vi "KN-AnnulusToArray.vi"(10 "Rectangle":T1 {"Rotation" format="%.2f"; "Left" scale=0.0..1024.0; "Right" scale=0.0..1024.0}, 11 "Annulus":T2 {"End Angle" format="%.2f"; "Start Angle" format="%.2f"; "Center X" scale=0.0..1024.0}) -> (2 "矩形":string, 3 "字符串":string)   [LabVIEW 2015]
panel:
  out "添加的数组":string[](array[string])
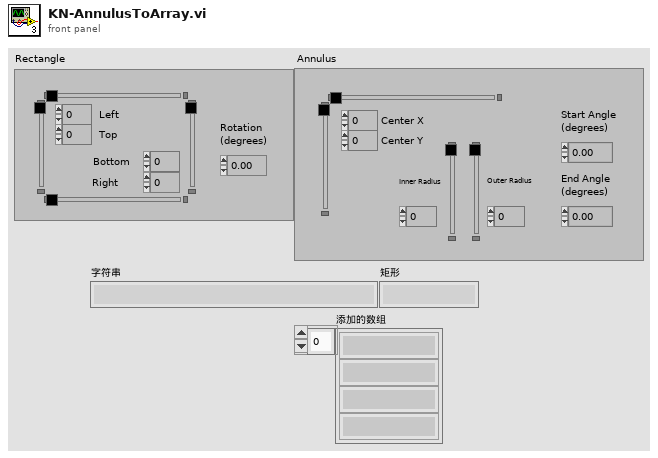
[diagram p1: front panel]
types:
  T1 = typedef "IMAQ Rectangle" = cluster{"Left":i32, "Top":i32, "Right":i32, "Bottom":i32, "Rotation":dbl}
  T2 = typedef "IMAQ Circle" = cluster{"Center X":i32, "Center Y":i32, "Inner Radius":i32, "Outer Radius":i32, "Start Angle":dbl, "End Angle":dbl}
  T3 = cluster{"Center X":string, "Center Y":string, "Inner Radius":string, "Outer Radius":string, "Start Angle":string, "End Angle":string}
  T4 = cluster{"Left":string, "Top":string, "Right":string, "Bottom":string, "Rotation":string}
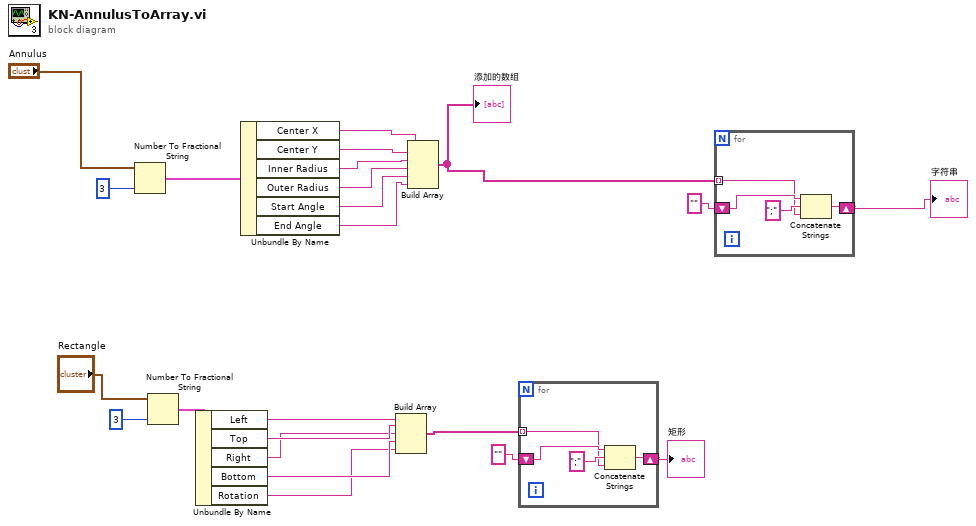
[diagram p0: block diagram]
diagram:
  n1 = Number To Fractional String(number="Annulus", precision (6)=i16 3 ("精度(6)")) -> (F-format string=w22:T3)  [unwired: 2 in]
  n2 = Number To Fractional String(number="Rectangle", precision (6)=i16 3 ("精度(6)")) -> (F-format string=w9:T4)  [unwired: 2 in]
  n3 = Unbundle By Name(w9) -> ("Left"=w8:string, "Top"=w7:string, "Right"=w6:string, "Bottom"=w5:string, "Rotation"=w4:string)
  n4 = Unbundle By Name(w22) -> ("Center X"=w21:string, "Center Y"=w20:string, "Inner Radius"=w19:string, "Outer Radius"=w18:string, "Start Angle"=w17:string, "End Angle"=w16:string)
  n5 = Build Array(w8, w7, w6, w5, w4) -> (w2:string[])
  n6 = Build Array(w21, w20, w19, w18, w17, w16) -> (w15:string[])
  "添加的数组" <- w15
  n7 = for {
    tunnel: w2 -> [w24] mode=indexing
    shift-right: [w27] -> w1
    shift-left: "" -> [w25]
    n8 = Concatenate Strings(w25, ";" ("字符串"), w24) -> (w27:string)
  }
  "矩形" <- w1
  n9 = for {
    tunnel: w15 -> [w28] mode=indexing
    shift-right: [w31] -> w12
    shift-left: "" -> [w29]
    n10 = Concatenate Strings(w29, ";" ("字符串"), w28) -> (w31:string)
  }
  "字符串" <- w12
